vi "Configure Measurement.vi"(8 "error in (no error)":errorcluster {"code" format="%.0x"}, 9 "Gating (False)":bool, 10 "Ref Lev Calc Method (Histogram)":i32(slide)=1, 11 "VISA Resource Name":refnum<visa-resource-name>) -> (0 "error out":errorcluster {"code" format="%.0x"}, 3 "VISA Resource Name Out":refnum<visa-resource-name>)   [LabVIEW 2010, in "Tektronix TDS 3000 Series.lvlib"]
doc: "This VI configures the method the oscilloscope uses to calculate the measurement reference levels, and controls whether the oscilloscope uses gating for measurements."
uses:
  <instrlib>/Tektronix TDS 3000 Series/Tektronix TDS 3000 Series.lvlib
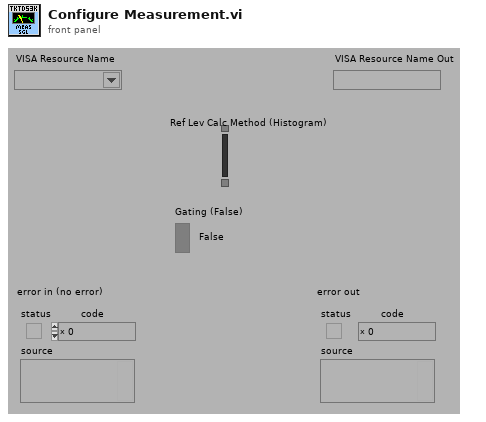
[diagram p1: front panel]
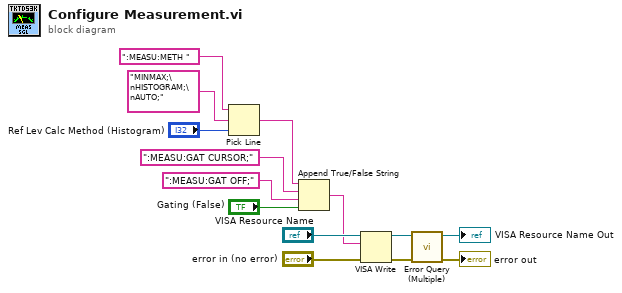
[diagram p0: block diagram]
diagram:
  n1 = Pick Line(string ("")=":MEASU:METH " ("multi-line string"), multi-line string="MINMAX;\nHISTOGRAM;\nAUTO;", line index="Ref Lev Calc Method (Histogram)") -> (output string=w7:string)
  n2 = Append True/False String(1:"Gating (False)", 2:":MEASU:GAT OFF;" ("false string"), 3:":MEASU:GAT CURSOR;" ("true string"), 4:w7) -> (0:w6:string)
  n3 = VISA Write(VISA resource name="VISA Resource Name", write buffer=w6, error in (no error)="error in (no error)") -> (VISA resource name out=w4:refnum<visa-resource-name>, error out=w3:errorcluster)  [unwired: 1 out]
  n4 = call <instrlib>:"Error Query (Multiple).vi"("error in (no error)"=w3, "VISA Resource Name"=w4) -> ("error out"=→"error out":errorcluster, "VISA Resource Name Out"=→"VISA Resource Name Out":refnum<visa-resource-name>)  [unwired: 6 in, 2 out]
